vi "Lab Panel V5.27.vi"() -> ()   [LabVIEW 2013] (continued)
                            n1774 = Bundle(cluster=w3324) -> (w3325:T4)  [unwired: 3 in]
                            n1775 = local write "RUN LAB05-2"(w3322) -> ()
                            n1776 = local write "O/I  LAB05-2"(w3322) -> ()
                            n1777 = local write "run lab05-2"(w3322) -> ()
                            n1778 = local write "DISP LAB05-2"(w3325) -> ()
                          }
                          frame #1 {
                            n1779 = TDMS Close(11:w3326) -> (0:w3327:errorcluster)  [unwired: 1 in, 1 out]
                            n1780 = local write "data file error"(w3327) -> ()
                          }
                          frame #2 {
                            n1781 = stacked-sequence {
                              tunnel: "LAB05-2" -> [w3335 w3341]
                              tunnel: w3332 -> [_ w3340]
                              tunnel: w3331 -> [_ w3339]
                              tunnel: w3330 -> [_ w3338]
                              tunnel: w3329 -> [_ w3337]
                              tunnel: w3328 -> [_ w3336]
                              frame #0 {
                                n1782 = call "sub vi - defrag tdms v1.vi"("panel id"=w3335) -> ("error out"=w3334:errorcluster)  [unwired: 10 in]
                                n1783 = local write "data file error"(w3334) -> ()
                              }
                              frame #1 {
                                n1784 = Bundle("STATUS"=w3340, "OUT SERVER ADDRESS"=w3339, "FROM ACCOUNT"=w3338, "Mail Test File To:"=w3337, "Mail Test Fail"=w3336) -> (w3343:T26)  [unwired: 1 in]
                                n1785 = call "Save data file (pass-fail) v5.vi"("Input Cluster"=w3343, "panel id"=w3341) -> ("network file save error"=w3342:errorcluster)  [unwired: 8 in, 1 out]
                                n1786 = local write "data file error"(w3342) -> ()
                              }
                            }
                          }
                        }
                      }
                    }
                  }
                }
              }
            }
            n1787 = global write "Global display 2.vi" "Mail test file to:"(w2851) -> ()
            n1788 = local read "Network Directory"() -> (w2857:path)
            n1789 = global write "Global 1.vi" "Network Drive"(w2857) -> ()
          }
          frame #8 {
            # "disable functions"
            n1790 = stacked-sequence {
              tunnel: w3353 -> [w3367 _ w3424]
              tunnel: w3352 -> [w3362 _ w3423]
              tunnel: w3351 -> [w3361 _ w3422]
              tunnel: w3350 -> [w3359 _ w3421]
              tunnel: w3349 -> [w3360 _ w3420]
              tunnel: w3348 -> [_ w3384 w3419]
              tunnel: w3347 -> [_ w3385 w3418]
              tunnel: w3346 -> [_ w3386 w3417]
              tunnel: w3345 -> [_ w3387 w3416]
              tunnel: w3344 -> [_ w3388 w3415]
              frame #0 {
                n1791 = Select(t=2, s=w3359, f=0) -> (s? t:f=w3355:i32)
                n1792 = Select(t=2, s=w3361, f=0) -> (s? t:f=w3356:i32)
                n1793 = Select(t=2, s=w3360, f=0) -> (s? t:f=w3354:i32)
                n1794 = Select(t=2, s=w3367, f=0) -> (s? t:f=w3358:i32)
                n1795 = Select(t=2, s=w3362, f=0) -> (s? t:f=w3357:i32)
                n1796 = property on="SELECT LAB02-2" class="RadioBtnsControl (strict)"("DisabledEnum"=w3355) -> ()  [unwired: 2 in, 2 out]
                n1797 = property on="SELECT LAB02-1" class="RadioBtnsControl (strict)"("DisabledEnum"=w3356) -> ()  [unwired: 2 in, 2 out]
                n1798 = property on="SELECT LAB03-1" class="RadioBtnsControl (strict)"("DisabledEnum"=w3354) -> ()  [unwired: 2 in, 2 out]
                n1799 = property on="SELECT LAB01-1" class="RadioBtnsControl (strict)"("DisabledEnum"=w3358) -> ()  [unwired: 2 in, 2 out]
                n1800 = property on="SELECT LAB01-2" class="RadioBtnsControl (strict)"("DisabledEnum"=w3357) -> ()  [unwired: 2 in, 2 out]
                n1801 = Not(x=w3367) -> (.not. x?=w3368:bool)
                n1802 = property on="RESULT LAB01-1" class="Bool (strict)"("Visible"=w3368) -> ()  [unwired: 2 in, 2 out]
                n1803 = Not(x=w3362) -> (.not. x?=w3366:bool)
                n1804 = Not(x=w3361) -> (.not. x?=w3365:bool)
                n1805 = Not(x=w3359) -> (.not. x?=w3364:bool)
                n1806 = property on="RESULT LAB01-2" class="Bool (strict)"("Visible"=w3366) -> ()  [unwired: 2 in, 2 out]
                n1807 = Not(x=w3360) -> (.not. x?=w3363:bool)
                n1808 = property on="RESULT LAB02-1" class="Bool (strict)"("Visible"=w3365) -> ()  [unwired: 2 in, 2 out]
                n1809 = property on="RESULT LAB02-2" class="Bool (strict)"("Visible"=w3364) -> ()  [unwired: 2 in, 2 out]
                n1810 = property on="RESULT LAB03-1" class="Bool (strict)"("Visible"=w3363) -> ()  [unwired: 2 in, 2 out]
                n1811 = property on="SET LAB01-1" class="Clust (strict)"("DisabledEnum"=w3358) -> ()  [unwired: 2 in, 2 out]
                n1812 = property on="SET LAB01-2" class="Clust (strict)"("DisabledEnum"=w3357) -> ()  [unwired: 2 in, 2 out]
                n1813 = property on="SET LAB02-1" class="Clust (strict)"("DisabledEnum"=w3356) -> ()  [unwired: 2 in, 2 out]
                n1814 = property on="SET LAB02-2" class="Clust (strict)"("DisabledEnum"=w3355) -> ()  [unwired: 2 in, 2 out]
                n1815 = property on="SET LAB03-1" class="Clust (strict)"("DisabledEnum"=w3354) -> ()  [unwired: 2 in, 2 out]
                n1816 = property on="O/I  LAB01-1" class="Bool (strict)"("DisabledEnum"=w3358) -> ()  [unwired: 2 in, 2 out]
                n1817 = property on="O/I  LAB01-2" class="Bool (strict)"("DisabledEnum"=w3357) -> ()  [unwired: 2 in, 2 out]
                n1818 = property on="O/I  LAB02-1" class="Bool (strict)"("DisabledEnum"=w3356) -> ()  [unwired: 2 in, 2 out]
                n1819 = property on="O/I  LAB02-2" class="Bool (strict)"("DisabledEnum"=w3355) -> ()  [unwired: 2 in, 2 out]
                n1820 = property on="O/I  LAB03-1" class="Bool (strict)"("DisabledEnum"=w3354) -> ()  [unwired: 2 in, 2 out]
              }
              frame #1 {
                n1821 = Select(t=2, s=w3388, f=0) -> (s? t:f=w3379:i32)
                n1822 = Select(t=2, s=w3387, f=0) -> (s? t:f=w3380:i32)
                n1823 = Select(t=2, s=w3384, f=0) -> (s? t:f=w3383:i32)
                n1824 = Select(t=2, s=w3385, f=0) -> (s? t:f=w3382:i32)
                n1825 = Select(t=2, s=w3386, f=0) -> (s? t:f=w3381:i32)
                n1826 = property on="SELECT LAB05-2" class="RadioBtnsControl (strict)"("DisabledEnum"=w3379) -> ()  [unwired: 2 in, 2 out]
                n1827 = property on="SELECT LAB05-1" class="RadioBtnsControl (strict)"("DisabledEnum"=w3380) -> ()  [unwired: 2 in, 2 out]
                n1828 = property on="SELECT LAB03-2" class="RadioBtnsControl (strict)"("DisabledEnum"=w3383) -> ()  [unwired: 2 in, 2 out]
                n1829 = property on="SELECT LAB04-1" class="RadioBtnsControl (strict)"("DisabledEnum"=w3382) -> ()  [unwired: 2 in, 2 out]
                n1830 = property on="SELECT LAB04-2" class="RadioBtnsControl (strict)"("DisabledEnum"=w3381) -> ()  [unwired: 2 in, 2 out]
                n1831 = property on="SET LAB05-2" class="Clust (strict)"("DisabledEnum"=w3379) -> ()  [unwired: 2 in, 2 out]
                n1832 = property on="SET LAB05-1" class="Clust (strict)"("DisabledEnum"=w3380) -> ()  [unwired: 2 in, 2 out]
                n1833 = property on="SET LAB03-2" class="Clust (strict)"("DisabledEnum"=w3383) -> ()  [unwired: 2 in, 2 out]
                n1834 = property on="SET LAB04-1" class="Clust (strict)"("DisabledEnum"=w3382) -> ()  [unwired: 2 in, 2 out]
                n1835 = property on="SET LAB04-2" class="Clust (strict)"("DisabledEnum"=w3381) -> ()  [unwired: 2 in, 2 out]
                n1836 = property on="O/I  LAB05-2" class="Bool (strict)"("DisabledEnum"=w3379) -> ()  [unwired: 2 in, 2 out]
                n1837 = property on="O/I  LAB05-1" class="Bool (strict)"("DisabledEnum"=w3380) -> ()  [unwired: 2 in, 2 out]
                n1838 = property on="O/I  LAB04-1" class="Bool (strict)"("DisabledEnum"=w3382) -> ()  [unwired: 2 in, 2 out]
                n1839 = property on="O/I  LAB04-2" class="Bool (strict)"("DisabledEnum"=w3381) -> ()  [unwired: 2 in, 2 out]
                n1840 = property on="O/I  LAB03-2" class="Bool (strict)"("DisabledEnum"=w3383) -> ()  [unwired: 2 in, 2 out]
                n1841 = Not(x=w3388) -> (.not. x?=w3389:bool)
                n1842 = Not(x=w3387) -> (.not. x?=w3390:bool)
                n1843 = Not(x=w3386) -> (.not. x?=w3391:bool)
                n1844 = property on="RESULT LAB05-2" class="Bool (strict)"("Visible"=w3389) -> ()  [unwired: 2 in, 2 out]
                n1845 = property on="RESULT LAB05-1" class="Bool (strict)"("Visible"=w3390) -> ()  [unwired: 2 in, 2 out]
                n1846 = Not(x=w3385) -> (.not. x?=w3392:bool)
                n1847 = property on="RESULT LAB04-2" class="Bool (strict)"("Visible"=w3391) -> ()  [unwired: 2 in, 2 out]
                n1848 = Not(x=w3384) -> (.not. x?=w3393:bool)
                n1849 = property on="RESULT LAB04-1" class="Bool (strict)"("Visible"=w3392) -> ()  [unwired: 2 in, 2 out]
                n1850 = property on="RESULT LAB03-2" class="Bool (strict)"("Visible"=w3393) -> ()  [unwired: 2 in, 2 out]
              }
              frame #2 {
                # "disable calibrate if any test running"
                n1851 = Or(x=w3416, y=w3415) -> (x .or. y?=w3409:bool)
                n1852 = Or(x=w3418, y=w3417) -> (x .or. y?=w3411:bool)
                n1853 = Or(x=w3422, y=w3421) -> (x .or. y?=w3413:bool)
                n1854 = Or(x=w3420, y=w3419) -> (x .or. y?=w3412:bool)
                n1855 = Or(x=w3424, y=w3423) -> (x .or. y?=w3414:bool)
                n1856 = Or(x=w3412, y=w3411) -> (x .or. y?=w3410:bool)
                n1857 = Or(x=w3414, y=w3413) -> (x .or. y?=w3408:bool)
                n1858 = Or(x=w3410, y=w3409) -> (x .or. y?=w3407:bool)
                n1859 = Or(x=w3408, y=w3407) -> (x .or. y?=w3404:bool)
                "Any Test Running" <- w3404
                n1860 = case shown="False" w3404 {
                  tunnel: [0 2] -> w3406
                  frame False {
                  }
                  frame True {
                  }
                }
                n1861 = property on="JIG TEST" class="Clust (strict)"("DisabledEnum"=w3406) -> ()  [unwired: 2 in, 2 out]
                n1862 = property on="Network Directory" class="Path"("DisabledEnum"=w3406) -> ()  [unwired: 2 in, 2 out]
                n1863 = property on="MAIL SETTINGS" class="Clust (strict)"("DisabledEnum"=w3406) -> ()  [unwired: 2 in, 2 out]
                n1864 = property on="SET (cal)" class="Bool (strict)"("DisabledEnum"=w3406) -> ()  [unwired: 2 in, 2 out]
                n1865 = property on="ADMIN" class="Bool (strict)"("DisabledEnum"=0) -> ()  [unwired: 2 in, 2 out]
              }
            }
          }
          frame #9 {
            # "drive jigs"
            n1866 = stacked-sequence {
              frame #0 {
                # "jig on"
                n1867 = local read "jig cycle"() -> (w3432:dbl)
                n1868 = property on="JIG TEST" class="Clust (strict)"() -> ("DisabledEnum"=w3429:T16)  [unwired: 2 in, 2 out]
                n1869 = Equal?(x=w3429, y=2) -> (x = y?=w3428:bool)
                n1870 = Equal?(x=w3432, y=0) -> (x = y?=w3430:bool)
                n1871 = And(x=w3430, y=w3428) -> (x .and. y?=w3427:bool)
                n1872 = case shown="True" w3427 {
                  frame False {
                  }
                  frame True {
                    n1873 = local read "run lab01-1"() -> (w3443:bool)
                    n1874 = local read "run lab01-2"() -> (w3442:bool)
                    n1875 = local read "run lab02-1"() -> (w3441:bool)
                    n1876 = local read "run lab02-2"() -> (w3440:bool)
                    n1877 = local read "run lab03-1"() -> (w3439:bool)
                    n1878 = local read "run lab03-2"() -> (w3438:bool)
                    n1879 = local read "run lab04-1"() -> (w3437:bool)
                    n1880 = local read "run lab04-2"() -> (w3436:bool)
                    n1881 = local read "run lab05-1"() -> (w3435:bool)
                    n1882 = local read "run lab05-2"() -> (w3434:bool)
                    n1883 = local write "JIG LAB03-2"(w3438) -> ()
                    n1884 = local write "JIG LAB01-1"(w3443) -> ()
                    n1885 = local write "JIG LAB01-2"(w3442) -> ()
                    n1886 = local write "JIG LAB02-1"(w3441) -> ()
                    n1887 = local write "JIG LAB02-2"(w3440) -> ()
                    n1888 = local write "JIG LAB03-1"(w3439) -> ()
                    n1889 = local write "JIG LAB04-1"(w3437) -> ()
                    n1890 = local write "JIG LAB04-2"(w3436) -> ()
                    n1891 = local write "JIG LAB05-1"(w3435) -> ()
                    n1892 = local write "JIG LAB05-2"(w3434) -> ()
                  }
                }
              }
              frame #1 {
                # "jig off"
                n1893 = local read "jig cycle"() -> (w3450:dbl)
                n1894 = local read "on loops"() -> (w3449:dbl)
                n1895 = property on="JIG TEST" class="Clust (strict)"() -> ("DisabledEnum"=w3448:T16)  [unwired: 2 in, 2 out]
                n1896 = Equal?(x=w3448, y=2) -> (x = y?=w3446:bool)
                n1897 = Equal?(x=w3450, y=w3449) -> (x = y?=w3445:bool)
                n1898 = And(x=w3445, y=w3446) -> (x .and. y?=w3444:bool)
                n1899 = case shown="True" w3444 {
                  frame False {
                  }
                  frame True {
                    w3501 = FALSE
                    w3502 = TRUE
                    w3500 = 2
                    n1900 = local read "SELECT LAB05-2"() -> (w3491:T3)
                    n1901 = local read "SELECT LAB04-2"() -> (w3493:T3)
                    n1902 = local read "SELECT LAB04-1"() -> (w3494:T3)
                    n1903 = local read "SELECT LAB05-1"() -> (w3492:T3)
                    n1904 = local read "SELECT LAB03-2"() -> (w3495:T3)
                    n1905 = local read "SELECT LAB02-1"() -> (w3498:T3)
                    n1906 = local read "SELECT LAB03-1"() -> (w3496:T3)
                    n1907 = local read "SELECT LAB02-2"() -> (w3497:T3)
                    n1908 = local read "SELECT LAB01-2"() -> (w3499:T3)
                    n1909 = local read "run lab05-1"() -> (w3461:bool)
                    n1910 = local read "run lab05-2"() -> (w3460:bool)
                    n1911 = local read "SELECT LAB01-1"() -> (w3503:T3)
                    n1912 = local read "run lab04-2"() -> (w3462:bool)
                    n1913 = local read "run lab04-1"() -> (w3463:bool)
                    n1914 = local read "run lab01-1"() -> (w3479:bool)
                    n1915 = local read "run lab01-2"() -> (w3468:bool)
                    n1916 = local read "run lab03-2"() -> (w3464:bool)
                    n1917 = local read "run lab03-1"() -> (w3465:bool)
                    n1918 = local read "run lab02-1"() -> (w3467:bool)
                    n1919 = local read "run lab02-2"() -> (w3466:bool)
                    n1920 = Equal?(x=w3500, y=w3496) -> (x = y?=w3474:bool)
                    n1921 = Equal?(x=w3500, y=w3495) -> (x = y?=w3473:bool)
                    n1922 = Equal?(x=w3500, y=w3494) -> (x = y?=w3472:bool)
                    n1923 = Equal?(x=w3500, y=w3493) -> (x = y?=w3471:bool)
                    n1924 = Equal?(x=w3500, y=w3492) -> (x = y?=w3470:bool)
                    n1925 = Equal?(x=w3500, y=w3491) -> (x = y?=w3469:bool)
                    n1926 = Equal?(x=w3500, y=w3503) -> (x = y?=w3480:bool)
                    n1927 = Equal?(x=w3500, y=w3498) -> (x = y?=w3476:bool)
                    n1928 = Equal?(x=w3500, y=w3497) -> (x = y?=w3475:bool)
                    n1929 = Equal?(x=w3500, y=w3499) -> (x = y?=w3477:bool)
                    n1930 = And(x=w3471, y=w3462) -> (x .and. y?=w3453:bool)
                    n1931 = And(x=w3474, y=w3465) -> (x .and. y?=w3456:bool)
                    n1932 = And(x=w3472, y=w3463) -> (x .and. y?=w3454:bool)
                    n1933 = And(x=w3469, y=w3460) -> (x .and. y?=w3451:bool)
                    n1934 = And(x=w3475, y=w3466) -> (x .and. y?=w3457:bool)
                    n1935 = And(x=w3473, y=w3464) -> (x .and. y?=w3455:bool)
                    n1936 = And(x=w3470, y=w3461) -> (x .and. y?=w3452:bool)
                    n1937 = And(x=w3477, y=w3468) -> (x .and. y?=w3459:bool)
                    n1938 = And(x=w3480, y=w3479) -> (x .and. y?=w3478:bool)
                    n1939 = And(x=w3476, y=w3467) -> (x .and. y?=w3458:bool)
                    n1940 = Select(t=w3502, s=w3478, f=w3501) -> (s? t:f=w3481:bool)
                    n1941 = Select(t=w3502, s=w3459, f=w3501) -> (s? t:f=w3482:bool)
                    n1942 = Select(t=w3502, s=w3458, f=w3501) -> (s? t:f=w3483:bool)
                    n1943 = Select(t=w3502, s=w3457, f=w3501) -> (s? t:f=w3484:bool)
                    n1944 = Select(t=w3502, s=w3456, f=w3501) -> (s? t:f=w3485:bool)
                    n1945 = Select(t=w3502, s=w3455, f=w3501) -> (s? t:f=w3486:bool)
                    n1946 = Select(t=w3502, s=w3454, f=w3501) -> (s? t:f=w3487:bool)
                    n1947 = Select(t=w3502, s=w3453, f=w3501) -> (s? t:f=w3488:bool)
                    n1948 = Select(t=w3502, s=w3452, f=w3501) -> (s? t:f=w3489:bool)
                    n1949 = Select(t=w3502, s=w3451, f=w3501) -> (s? t:f=w3490:bool)
                    n1950 = local write "JIG LAB03-2"(w3486) -> ()
                    n1951 = local write "JIG LAB02-1"(w3483) -> ()
                    n1952 = local write "JIG LAB02-2"(w3484) -> ()
                    n1953 = local write "JIG LAB01-2"(w3482) -> ()
                    n1954 = local write "JIG LAB03-1"(w3485) -> ()
                    n1955 = local write "JIG LAB01-1"(w3481) -> ()
                    n1956 = local write "JIG LAB05-2"(w3490) -> ()
                    n1957 = local write "JIG LAB04-1"(w3487) -> ()
                    n1958 = local write "JIG LAB05-1"(w3489) -> ()
                    n1959 = local write "JIG LAB04-2"(w3488) -> ()
                  }
                }
              }
            }
          }
          frame #10 {
            # "enable  jig test output if no test busy"
            n1960 = property on="JIG TEST" class="Clust (strict)"() -> ("DisabledEnum"=w3506:T16)  [unwired: 2 in, 2 out]
            n1961 = Equal?(x=w3506, y=0) -> (x = y?=w3504:bool)
            n1962 = case shown="True" w3504 {
              frame False {
              }
              frame True {
                n1963 = local read "JIG TEST"() -> (w3517:T10)
                n1964 = Unbundle(w3517) -> ("LAB01-1"=w3516:bool, "LAB01-2"=w3515:bool, "LAB02-1"=w3514:bool, "LAB02-2"=w3513:bool, "LAB03-1"=w3512:bool, "LAB03-2"=w3511:bool, "LAB04-1"=w3510:bool, "LAB04-2"=w3509:bool, "LAB05-1"=w3508:bool, "LAB05-2"=w3507:bool)
                n1965 = local write "JIG LAB05-1"(w3508) -> ()
                n1966 = local write "JIG LAB05-2"(w3507) -> ()
                n1967 = local write "JIG LAB04-1"(w3510) -> ()
                n1968 = local write "JIG LAB04-2"(w3509) -> ()
                n1969 = local write "JIG LAB03-2"(w3511) -> ()
                n1970 = local write "JIG LAB01-1"(w3516) -> ()
                n1971 = local write "JIG LAB02-1"(w3514) -> ()
                n1972 = local write "JIG LAB03-1"(w3512) -> ()
                n1973 = local write "JIG LAB01-2"(w3515) -> ()
                n1974 = local write "JIG LAB02-2"(w3513) -> ()
              }
            }
          }
          frame #11 {
            w3518 = FALSE
            # "Drive digital output and reset USB and temperature network if required."
            n1975 = global read "Global display 3.vi" "cycle O/F"() -> (w3527:bool)
            n1976 = local read "O/I  LAB05-2"() -> (w3520:bool)
            n1977 = local read "O/I  LAB05-1"() -> (w3522:bool)
            n1978 = local read "JIG LAB05-2"() -> (w3519:bool)
            n1979 = local read "O/I  LAB04-2"() -> (w3524:bool)
            n1980 = local read "JIG LAB05-1"() -> (w3521:bool)
            n1981 = local read "JIG LAB04-2"() -> (w3523:bool)
            n1982 = local read "O/I  LAB03-1"() -> (w3538:bool)
            n1983 = local read "O/I  LAB04-1"() -> (w3534:bool)
            n1984 = local read "O/I  LAB02-1"() -> (w3542:bool)
            n1985 = local read "O/I  LAB02-2"() -> (w3540:bool)
            n1986 = local read "O/I  LAB03-2"() -> (w3536:bool)
            n1987 = local read "JIG LAB04-1"() -> (w3533:bool)
            n1988 = local read "JIG LAB03-2"() -> (w3535:bool)
            n1989 = local read "O/I  LAB01-2"() -> (w3544:bool)
            n1990 = local read "JIG LAB02-1"() -> (w3541:bool)
            n1991 = local read "JIG LAB02-2"() -> (w3539:bool)
            n1992 = local read "JIG LAB03-1"() -> (w3537:bool)
            n1993 = local read "O/I  LAB01-1"() -> (w3546:bool)
            n1994 = local read "JIG LAB01-2"() -> (w3543:bool)
            n1995 = local read "JIG LAB01-1"() -> (w3545:bool)
            n1996 = case shown="False" w3527 {
              tunnel: [w3662 FALSE] -> w3526
              frame False {
                n1997 = local read "Analog error"() -> (w3664:bool)
                n1998 = local read "Reset Measuring"() -> (w3663:bool)
                n1999 = Or(x=w3663, y=w3664) -> (x .or. y?=w3662:bool)
              }
              frame True {
              }
            }
            n2000 = Build Array(w3539, w3538, w3537, w3536, w3535, w3534, w3533) -> (w3531:bool[])
            "USB OUT 1" <- w3531
            n2001 = Build Array(w3546, w3545, w3544, w3543, w3542, w3541, w3540) -> (w3532:bool[])
            "USB OUT 0" <- w3532
            n2002 = Build Array(w3524, w3523, w3522, w3521, w3520, w3519, w3518, w3518) -> (w3530:bool[])
            "USB OUT 2" <- w3530
            n2003 = Not(x=w3527) -> (.not. x?=w3528:bool)
            n2004 = local read "Simulate"() -> (w3529:bool)
            n2005 = And(x=w3528, y=w3526) -> (x .and. y?=w3525:bool)
            n2006 = stacked-sequence {
              tunnel: w3532 -> [w3550 w3556]
              tunnel: w3531 -> [w3549 w3555]
              tunnel: w3530 -> [w3548 w3554]
              tunnel: w3529 -> [w3547 w3557]
              tunnel: w3525 -> [_ w3558]
              frame #0 {
                # "drive outputs for normal use"
                n2007 = case shown="False" w3547 {
                  tunnel: w3550 -> [w3553 _]
                  tunnel: w3549 -> [w3552 _]
                  tunnel: w3548 -> [w3551 _]
                  frame False {
                    n2008 = call "sub vi - Drive Relays All v6.vi"("Array #2"=w3551, "Array #1"=w3552, "Array #0"=w3553) -> ()  [unwired: 8 in, 1 out]
                  }
                  frame True {
                  }
                }
              }
              frame #1 {
                # "USB  reset routine"
                n2009 = case shown="True" w3558 {
                  tunnel: w3557 -> [_ w3562]
                  tunnel: w3556 -> [_ w3561]
                  tunnel: w3555 -> [_ w3560]
                  tunnel: w3554 -> [_ w3559]
                  frame False {
                  }
                  frame True {
                    n2010 = stacked-sequence {
                      seq-local: [w3564 _ _ _ _] -> [_ w3570 _ _ _]
                      tunnel: w3562 -> [_ w3574 _ _ _]
                      tunnel: w3561 -> [_ w3573 _ _ _]
                      tunnel: w3560 -> [_ w3572 _ _ _]
                      tunnel: w3559 -> [_ w3571 _ _ _]
                      frame #0 {
                        n2011 = case shown="False" "Auto Reset" {
                          tunnel: [w3567 FALSE] -> w3565
                          frame False {
                            n2012 = Two Button Dialog(message="System reset") -> (T button?=w3567:bool)  [unwired: 2 in]
                          }
                          frame True {
                          }
                        }
                        n2013 = disable-structure shown="Disabled" {
                          frame Disabled {
                            n2014 = local write "Tab Control 2"(5) -> ()
                          }
                          frame Enabled {
                          }
                        }
                        n2015 = Or(x="Auto Reset", y=w3565) -> (x .or. y?=w3564:bool)
                      }
                      frame #1 {
                        n2016 = case shown="True" w3570 {
                          tunnel: w3574 -> [_ w3580]
                          tunnel: w3573 -> [_ w3579]
                          tunnel: w3572 -> [_ w3578]
                          tunnel: w3571 -> [_ w3577]
                          frame False {
                          }
                          frame True {
                            n2017 = stacked-sequence {
                              tunnel: w3580 -> [_ w3598 _]
                              tunnel: bool[] [] -> [w3583 w3597 w3619]
                              tunnel: w3579 -> [_ _ w3618]
                              tunnel: w3578 -> [w3582 _ w3617]
                              tunnel: w3577 -> [w3581 _ w3616]
                              tunnel: 5000 -> [w3584 _ w3615]
                              frame #0 {
                                # "switch off test stations for system reset"
                                n2018 = stacked-sequence {
                                tunnel: w3584 -> [w3588 w3592 w3594]
                                tunnel: w3583 -> [w3587 w3591 w3595]
                                tunnel: w3582 -> [w3586 _ _]
                                tunnel: w3581 -> [w3585 w3590 _]
                                frame #0 {
                                # "drive 1st 7 inputs"
                                n2019 = call "sub vi - Drive Relays All v6.vi"("Array #2"=w3585, "Array #1"=w3586, "Array #0"=w3587) -> ()  [unwired: 8 in, 1 out]
                                n2020 = call "Message Display V1.vi"("Message"="Delay off LAB 01-1 to 02-1", "Delay mS"=w3588) -> ()  [unwired: 10 in]
                                }
                                frame #1 {
                                # "drive 2nd 7 inputs"
                                n2021 = call "sub vi - Drive Relays All v6.vi"("Array #2"=w3590, "Array #1"=w3591, "Array #0"=w3591) -> ()  [unwired: 8 in, 1 out]
                                n2022 = call "Message Display V1.vi"("Message"="Delay off LAB 02-2 to 04-1", "Delay mS"=w3592) -> ()  [unwired: 10 in]
                                }
                                frame #2 {
                                # "drive 3rd 7 inputs"
                                n2023 = call "sub vi - Drive Relays All v6.vi"("Array #2"=w3595, "Array #1"=w3595, "Array #0"=w3595) -> ()  [unwired: 8 in, 1 out]
                                n2024 = call "Message Display V1.vi"("Message"="Delay off LAB 04-2 to 05-2", "Delay mS"=w3594) -> ()  [unwired: 10 in]
                                }
                                }
                              }
                              frame #1 {
                                # "reset all usb modules"
                                n2025 = stacked-sequence {
                                tunnel: w3598 -> [_ w3603]
                                tunnel: w3597 -> [w3601 _]
                                frame #0 {
                                n2026 = local write "AI Task"(FALSE) -> ()
                                n2027 = call "sub vi - Drive Relays All v6.vi"("Array #2"=bool[] [FALSE, FALSE, FALSE, FALSE, FALSE, FALSE, TRUE, FALSE], "Array #1"=w3601, "Array #0"=w3601) -> ()  [unwired: 8 in, 1 out]
                                }
                                frame #1 {
                                n2028 = call "Reset Meas v 5.vi"("simulate"=w3603) -> ("Reset Error"=w3602:bool)  [unwired: 10 in]
                                n2029 = case shown="False" w3602 {
                                frame False {
                                n2030 = local read "AI Task0"() -> (w3610:dbl)
                                n2031 = local read "AI Task1"() -> (w3609:dbl)
                                n2032 = local read "AI Task2"() -> (w3608:dbl)
                                n2033 = local read "RATE (Hz)"() -> (w3607:dbl)
                                n2034 = local read "SAMPLES"() -> (w3606:dbl)
                                n2035 = call "sub vi - AI USB4704 (3)  Create Task v3.vi"("Task In 0"=w3610, "Task In 1"=w3609, "Task In 2"=w3608, "Rate Hz"=w3607, "Samples"=w3606) -> ("TASK USB 0"=w3613:i32, "TASK USB 1"=w3612:i32, "TASK USB 2"=w3611:i32, "AI Task Er"=w3604:bool)  [unwired: 6 in, 1 out]
                                n2036 = local write "AI Task"(TRUE) -> ()
                                n2037 = local write "Reset Error"(w3604) -> ()
                                n2038 = local write "AI Task2"(w3611) -> ()
                                n2039 = local write "AI Task1"(w3612) -> ()
                                n2040 = local write "AI Task0"(w3613) -> ()
                                }
                                frame True {
                                "Reset Error" <- TRUE
                                }
                                }
                                }
                                }
                              }
                              frame #2 {
                                # "switch test stations back on after reset"
                                n2041 = stacked-sequence {
                                tunnel: w3619 -> [w3623 w3626 _]
                                tunnel: w3618 -> [w3622 w3628 w3633]
                                tunnel: w3615 -> [w3621 w3624 w3630]
                                tunnel: w3617 -> [_ w3627 w3632]
                                tunnel: w3616 -> [_ _ w3629]
                                frame #0 {
                                # "drive 1st 7 inputs"
                                n2042 = call "sub vi - Drive Relays All v6.vi"("Array #2"=w3623, "Array #1"=w3623, "Array #0"=w3622) -> ()  [unwired: 8 in, 1 out]
                                n2043 = call "Message Display V1.vi"("Message"="Delay on LAB 01-1 to 02-1", "Delay mS"=w3621) -> ()  [unwired: 10 in]
                                }
                                frame #1 {
                                # "drive 1st & 2nd outputs"
                                n2044 = call "sub vi - Drive Relays All v6.vi"("Array #2"=w3626, "Array #1"=w3627, "Array #0"=w3628) -> ()  [unwired: 8 in, 1 out]
                                n2045 = call "Message Display V1.vi"("Message"="Delay on LAB 02-2 to 04-1", "Delay mS"=w3624) -> ()  [unwired: 10 in]
                                }
                                frame #2 {
                                n2046 = call "sub vi - Drive Relays All v6.vi"("Array #2"=w3629, "Array #1"=w3632, "Array #0"=w3633) -> ()  [unwired: 8 in, 1 out]
                                n2047 = call "Message Display V1.vi"("Message"="Delay on LAB 04-2 to 05-2", "Delay mS"=w3630) -> ()  [unwired: 10 in]
                                }
                                }
                              }
                            }
                          }
                        }
                      }
                      frame #2 {
                        w3634 = 0
                        w3635 = FALSE
                        # "set all back to zero"
                        n2048 = local read "Total USB resets"() -> (w3637:dbl)
                        n2049 = local read "Resets Done"() -> (w3639:dbl)
                        n2050 = local write "Reset Measuring"(w3635) -> ()
                        n2051 = local write "Analog error"(w3635) -> ()
                        n2052 = local write "Er USB#2"(w3634) -> ()
                        n2053 = local write "Er USB#0"(w3634) -> ()
                        n2054 = local write "Er USB#1"(w3634) -> ()
                        n2055 = local write "Error USB #0"(w3635) -> ()
                        n2056 = local write "Error USB #1"(w3635) -> ()
                        n2057 = local write "Error USB #2"(w3635) -> ()
                        n2058 = Increment(x=w3637) -> (x+1=w3636:dbl)
                        n2059 = Increment(x=w3639) -> (x+1=→"Resets Done":dbl)
                        n2060 = local write "Total USB resets"(w3636) -> ()
                      }
                      frame #3 {
                        # "save reset value"
                        n2061 = String To Path(string="c:\\crabtree\\Set Up\\") -> (path=w3649:path)
                        n2062 = Build Path(base path=w3649, name or relative path="USB resets.bin") -> (appended path=w3642:path)
                        n2063 = Create Folder(path (use dialog)=w3649) -> (error out=w3641:errorcluster)  [unwired: 2 in, 2 out]
                        n2064 = local read "Total USB resets"() -> (w3640:dbl)
                        n2065 = call <vilib>:"Clear Errors.vi"("error in (no error)"=w3641) -> ()  [unwired: 6 in, 1 out]
                        n2066 = Open/Create/Replace File(file path (use dialog)=w3642, operation (0:open)=T17."replace or create") -> (refnum out=w3647:refnum<file>, error out=w3646:errorcluster)  [unwired: 4 in, 1 out]
                        n2067 = Write to Binary File(file (use dialog)=w3647, data=w3640, error in=w3646) -> (refnum out=w3645:refnum<file>, error out=w3644:errorcluster)  [unwired: 3 in, 1 out]
                        n2068 = Close File(refnum=w3645, error in=w3644) -> (error out=w3643:errorcluster)  [unwired: 1 out]
                        n2069 = local write "data file error"(w3643) -> ()
                      }
                      frame #4 {
                        # "mail reset value"
                        n2070 = local read "MAIL SETTINGS"() -> (w3655:T7)
                        n2071 = local read "Total USB resets"() -> (w3659:dbl)
                        n2072 = Unbundle(w3655) -> ("OUT SERVER ADDRESS"=w3661:string, "FROM ACCOUNT"=w3660:string)  [unwired: 5 out]
                        n2073 = Number To Decimal String(number=w3659) -> (decimal integer string=w3657:string)  [unwired: 1 in]
                        n2074 = Concatenate Strings("Total USB resets: ", w3657) -> (w3656:string)
                        n2075 = call "sub vi - send mail v5.vi"("TO:"="francois@ffg.net", "subject"=w3656, "from"=w3660, "out going server"=w3661) -> ("error out"=w3654:errorcluster)  [unwired: 11 in]
                        n2076 = Bundle(cluster=w3655, "mail error"=w3654) -> (w3653:T7)  [unwired: 6 in]
                        n2077 = local write "MAIL SETTINGS"(w3653) -> ()
                      }
                    }
                  }
                }
              }
            }
          }
          frame #12 {
            # "if all test panels are off stop analog read"
            n2078 = local read "O/I  LAB03-1"() -> (w3687:bool)
            n2079 = local read "O/I  LAB03-2"() -> (w3686:bool)
            n2080 = local read "O/I  LAB04-1"() -> (w3685:bool)
            n2081 = local read "O/I  LAB04-2"() -> (w3684:bool)
            n2082 = local read "O/I  LAB05-1"() -> (w3683:bool)
            n2083 = local read "O/I  LAB05-2"() -> (w3682:bool)
            n2084 = local read "O/I  LAB02-2"() -> (w3688:bool)
            n2085 = local read "O/I  LAB02-1"() -> (w3689:bool)
            n2086 = local read "O/I  LAB01-2"() -> (w3690:bool)
            n2087 = local read "O/I  LAB01-1"() -> (w3691:bool)
            n2088 = Or(x=w3683, y=w3682) -> (x .or. y?=w3680:bool)
            n2089 = Or(x=w3685, y=w3684) -> (x .or. y?=w3681:bool)
            n2090 = Or(x=w3689, y=w3688) -> (x .or. y?=w3679:bool)
            n2091 = Or(x=w3687, y=w3686) -> (x .or. y?=w3677:bool)
            n2092 = Or(x=w3691, y=w3690) -> (x .or. y?=w3678:bool)
            n2093 = Or(x=w3681, y=w3680) -> (x .or. y?=w3674:bool)
            n2094 = Or(x=w3678, y=w3679) -> (x .or. y?=w3676:bool)
            n2095 = Or(x=w3676, y=w3677) -> (x .or. y?=w3675:bool)
            n2096 = local read "Any Test Running"() -> (w3673:bool)
            n2097 = Or(x=w3675, y=w3674) -> (x .or. y?=w3672:bool)
            n2098 = local read "AI Task"() -> (w3668:bool)
            n2099 = Or(x=w3672, y=w3673) -> (x .or. y?=w3667:bool)
            n2100 = Not(x=w3667) -> (.not. x?=w3671:bool)
            n2101 = Not(x=w3668) -> (.not. x?=w3669:bool)
            n2102 = And(x=w3671, y=w3668) -> (x .and. y?=w3670:bool)
            n2103 = And(x=w3667, y=w3669) -> (x .and. y?=w3666:bool)
            n2104 = case shown="True" w3670 {
              frame False {
              }
              frame True {
                # "close task if no test"
                n2105 = stacked-sequence {
                  seq-local: [w3705 _] -> [_ w3716]
                  frame #0 {
                    # "send mail of test cycle values"
                    n2106 = local read "JIG RELAY CYCLES"() -> (w3709:T8)
                    n2107 = Cluster To Array(cluster=w3709) -> (array=w3706:dbl[])
                    n2108 = Reverse 1D Array(array=w3706) -> (reversed array=w3707:dbl[])
                    n2109 = for {
                      tunnel: w3707 -> [w3714] mode=indexing
                      shift-right: [w3712] -> w3705
                      shift-left: "" -> [w3711]
                      n2110 = Number To Decimal String(number=w3714) -> (decimal integer string=w3713:string)  [unwired: 1 in]
                      n2111 = Concatenate Strings(w3713, ":", w3711) -> (w3712:string)
                    }
                  }
                  frame #1 {
                    n2112 = local read "MAIL SETTINGS"() -> (w3718:T7)
                    n2113 = Unbundle(w3718) -> ("OUT SERVER ADDRESS"=w3719:string, "FROM ACCOUNT"=w3720:string)  [unwired: 5 out]
                    n2114 = Concatenate Strings("Test Cycles:", w3716) -> (w3722:string)
                    n2115 = call "sub vi - send mail v5.vi"("TO:"="francois@ffg.net", "subject"=w3722, "Info"="Jig total cycle values", "from"=w3720, "out going server"=w3719) -> ("error out"=w3723:errorcluster)  [unwired: 10 in]
                    n2116 = Bundle(cluster=w3718, "mail error"=w3723) -> (w3717:T7)  [unwired: 6 in]
                    n2117 = local write "MAIL SETTINGS"(w3717) -> ()
                  }
                }
                n2118 = local read "AI Task2"() -> (w3704:dbl)
                n2119 = local read "AI Task1"() -> (w3703:dbl)
                n2120 = local read "AI Task0"() -> (w3702:dbl)
                n2121 = local write "AI Task"(FALSE) -> ()
                n2122 = call "sub vi - AI USB4704 (3)  Close Task v1.vi"("TASK USB 0"=w3702, "TASK USB 1"=w3703, "TASK USB 2"=w3704) -> ()  [unwired: 13 in]
              }
            }
            n2123 = case shown="True" w3666 {
              frame False {
              }
              frame True {
                # "create task for test"
                n2124 = local read "SAMPLES"() -> (w3696:dbl)
                n2125 = local read "RATE (Hz)"() -> (w3695:dbl)
                n2126 = local read "AI Task2"() -> (w3694:dbl)
                n2127 = local read "AI Task0"() -> (w3692:dbl)
                n2128 = local read "AI Task1"() -> (w3693:dbl)
                n2129 = call "sub vi - AI USB4704 (3)  Create Task v3.vi"("Task In 0"=w3692, "Task In 1"=w3693, "Task In 2"=w3694, "Rate Hz"=w3695, "Samples"=w3696) -> ("TASK USB 0"=w3697:i32, "TASK USB 1"=w3698:i32, "TASK USB 2"=w3699:i32)  [unwired: 6 in, 2 out]
                n2130 = local write "AI Task0"(w3697) -> ()
                n2131 = local write "AI Task1"(w3698) -> ()
                n2132 = local write "AI Task2"(w3699) -> ()
                n2133 = local write "AI Task"(TRUE) -> ()
              }
            }
          }
          frame #13 {
            # "get all analog values from USB devices"
            n2134 = local read "on loops"() -> (w3732:dbl)
            n2135 = local read "jig cycle"() -> (w3729:dbl)
            n2136 = Add(x=w3732, y=3) -> (x+y=w3730:dbl)
            n2137 = Equal?(x=w3729, y=3) -> (x = y?=w3727:bool)
            n2138 = Equal?(x=w3729, y=w3730) -> (x = y?=w3728:bool)
            n2139 = Or(x=w3727, y=w3728) -> (x .or. y?=w3726:bool)
            n2140 = global write "Global display 3.vi" "cycle O/F"(w3727) -> ()
            n2141 = case shown="True" w3726 {
              tunnel: w3727 -> [_ w3738]
              tunnel: w3725 -> [_ w3735]
              frame False {
              }
              frame True {
                n2142 = local read "Simulate"() -> (w3741:bool)
                n2143 = case shown="False" w3741 {
                  tunnel: [w3757 dynamicdata[] [] ("array GRAPH")] -> w3747
                  tunnel: [w3756 w3782] -> w3746
                  tunnel: [w3755 w3782] -> w3745
                  tunnel: [w3754 w3782] -> w3744
                  tunnel: [w3753 w3782] -> w3743
                  tunnel: [w3752 w3782] -> w3742
                  tunnel: w3738 -> [_ w3786]
                  tunnel: [w3751 "Ambient Volts"] -> w3737
                  tunnel: [w3750 bool[] []] -> w3736
                  tunnel: w3735 -> [w3749 _]
                  tunnel: [w3748 0.3 ("Analog loop time")] -> w3734
                  frame False {
                    # "analog in"
                    n2144 = case shown="True" w3749 {
                      tunnel: [dynamicdata[] [] ("array GRAPH") w3776] -> w3757
                      tunnel: [w3759 w3775] -> w3756
                      tunnel: [w3759 w3774] -> w3755
                      tunnel: [w3759 w3773] -> w3754
                      tunnel: [w3759 w3772] -> w3753
                      tunnel: [w3759 w3771] -> w3752
                      tunnel: [3 w3770] -> w3751
                      tunnel: [bool[] [] w3769] -> w3750
                      tunnel: [0.0 w3765] -> w3748
                      frame False {
                        w3760 = 0.0
                        # "no test"
                        n2145 = Bundle(w3760, w3760, w3760, w3760, w3760, w3760) -> (w3759:cluster{dbl, dbl, dbl, dbl, dbl, dbl})  [unwired: 1 in]
                      }
                      frame True {
                        # "test on"
                        n2146 = local read "AI data 0"() -> (w3768:waveform(dbl)[])
                        n2147 = local read "AI data 1"() -> (w3767:waveform(dbl)[])
                        n2148 = local read "AI data 2"() -> (w3764:waveform(dbl)[])
                        n2149 = local read "AI Error"() -> (w3766:errorcluster[])
                        n2150 = call "sub vi - Read Analog All v9.5.vi"("data 0"=w3768, "data 1"=w3767, "data 2"=w3764, "AI Error"=w3766) -> ("array GRAPH"=w3776:dynamicdata[], "LAB01"=w3775:T27, "LAB02"=w3774:T28, "LAB03"=w3773:T29, "LAB04"=w3772:T30, "deg C"=w3770:dbl, "USB Error"=w3769:bool[], "LAB05"=w3771:T31)  [unwired: 4 in]
                        n2151 = local read "AI loop time"() -> (w3765:dbl)
                      }
                    }
                  }
                  frame True {
                    # "simulate"
                    n2152 = local read "ON amps"() -> (w3780:dbl)
                    n2153 = local read "OFF amps"() -> (w3781:dbl)
                    n2154 = local read "VOLTS"() -> (w3784:dbl)
                    n2155 = local read "PF"() -> (w3783:dbl)
                    n2156 = Select(t=w3780, s=w3786, f=w3781) -> (s? t:f=w3785:dbl)
                    n2157 = Bundle("OFF amps"=w3785, "VOLTS"=w3784, "PF"=w3783, "OFF amps"=w3785, "VOLTS"=w3784, "PF"=w3783) -> (w3782:T32)  [unwired: 1 in]
                  }
                }
                n2158 = local read "Simulate"() -> (w3740:bool)
                n2159 = stacked-sequence {
                  seq-local: [w3790 _ _ _ _ _ _ _] -> [_ _ _ _ _ _ _ _]
                  seq-local: [w3789 _ _ _ _ _ _ _] -> [_ _ _ _ _ _ _ _]
                  seq-local: [w3788 _ _ _ _ _ _ _] -> [_ _ _ _ _ _ _ w3983]
                  tunnel: w3747 -> [_ w3841 _ _ _ _ _ _]
                  tunnel: w3746 -> [_ _ w3868 _ _ _ _ _]
                  tunnel: w3745 -> [_ _ _ w3896 _ _ _ _]
                  tunnel: w3744 -> [_ _ _ _ w3924 _ _ _]
                  tunnel: w3743 -> [_ _ _ _ _ w3952 _ _]
                  tunnel: w3742 -> [_ _ _ _ _ _ w3980 _]
                  tunnel: w3740 -> [_ _ w3867 w3895 w3923 w3951 w3979 w3985]
                  tunnel: T14 {"1  (A) cal"=1.0, "1 (V) cal"=1.0, "1 (PF) cal"=1.0, "1 (TL) cal"=1.0, "1 (TN) cal"=1.0, "2 (A) cal"=1.0, "2 (V) cal"=1.0, "2 (PF) cal"=1.0, "2 (TL) cal"=1.0, "2 (TN) cal"=1.0} ("CAL LAB01") -> [_ _ w3866 w3894 w3922 w3950 w3978 _]
                  tunnel: w3737 -> [_ _ _ _ _ _ _ w3984]
                  tunnel: w3736 -> [w3793 _ _ _ _ _ _ _]
                  tunnel: w3734 -> [_ w3820 _ _ _ _ _ _]
                  frame #0 {
                    n2160 = Index Array(array=w3793, index=2) -> (element=w3788:bool)
                    n2161 = Index Array(array=w3793, index=1) -> (element=w3789:bool)
                    n2162 = Index Array(array=w3793, index=0) -> (element=w3790:bool)
                    n2163 = local write "Error USB #2"(w3788) -> ()
                    n2164 = local write "Error USB #0"(w3790) -> ()
                    n2165 = local write "Error USB #1"(w3789) -> ()
                    n2166 = stacked-sequence {
                      tunnel: w3790 -> [w3797 _ _ _]
                      tunnel: w3789 -> [_ w3802 _ _]
                      tunnel: 0 -> [w3796 w3801 w3806 _]
                      tunnel: w3788 -> [_ _ w3807 _]
                      frame #0 {
                        n2167 = case shown="True" w3797 {
                          tunnel: w3796 -> [w3798 _]
                          frame False {
                            n2168 = local write "Er USB#0"(w3798) -> ()
                          }
                          frame True {
                            n2169 = local read "Er USB#0"() -> (w3800:dbl)
                            n2170 = Increment(x=w3800) -> (x+1=→"Er USB#0":dbl)
                          }
                        }
                      }
                      frame #1 {
                        n2171 = case shown="True" w3802 {
                          tunnel: w3801 -> [w3803 _]
                          frame False {
                            n2172 = local write "Er USB#1"(w3803) -> ()
                          }
                          frame True {
                            n2173 = local read "Er USB#1"() -> (w3805:dbl)
                            n2174 = Increment(x=w3805) -> (x+1=→"Er USB#1":dbl)
                          }
                        }
                      }
                      frame #2 {
                        n2175 = case shown="True" w3807 {
                          tunnel: w3806 -> [w3808 _]
                          frame False {
                            n2176 = local write "Er USB#2"(w3808) -> ()
                          }
                          frame True {
                            n2177 = local read "Er USB#2"() -> (w3810:dbl)
                            n2178 = Increment(x=w3810) -> (x+1=→"Er USB#2":dbl)
                          }
                        }
                      }
                      frame #3 {
                        w3816 = 10
                        n2179 = local read "Er USB#2"() -> (w3817:dbl)
                        n2180 = local read "Er USB#0"() -> (w3819:dbl)
                        n2181 = local read "Er USB#1"() -> (w3818:dbl)
                        n2182 = Greater Or Equal?(x=w3819, y=w3816) -> (x >= y?=w3814:bool)
                        n2183 = Greater Or Equal?(x=w3818, y=w3816) -> (x >= y?=w3813:bool)
                        n2184 = Greater Or Equal?(x=w3817, y=w3816) -> (x >= y?=w3812:bool)
                        n2185 = Or(x=w3814, y=w3813) -> (x .or. y?=w3815:bool)
                        n2186 = Or(x=w3815, y=w3812) -> (x .or. y?=→"Analog error":bool)
                      }
                    }
                  }
                  frame #1 {
                    # "display graph data on ADM page"
                    n2187 = local write "AI loop time"(w3820) -> ()
                    n2188 = local write "AI"(TRUE) -> ()
                    n2189 = Index Array(array=w3841, index=6) -> (element=→"LAB04-1 (GRAPH)":dynamicdata)
                    n2190 = Index Array(array=w3841, index=7) -> (element=→"LAB04-2 (GRAPH)":dynamicdata)
                    n2191 = Index Array(array=w3841, index=9) -> (element=→"LAB05-2 (GRAPH)":dynamicdata)
                    n2192 = Index Array(array=w3841, index=8) -> (element=→"LAB05-1 (GRAPH)":dynamicdata)
                    n2193 = Index Array(array=w3841, index=5) -> (element=→"LAB03-2 (GRAPH)":dynamicdata)
                    n2194 = Index Array(array=w3841, index=0) -> (element=→"LAB01-1 (GRAPH)":dynamicdata)
                    n2195 = Index Array(array=w3841, index=1) -> (element=→"LAB01-2 (GRAPH)":dynamicdata)
                    n2196 = Index Array(array=w3841, index=2) -> (element=→"LAB02-1 (GRAPH)":dynamicdata)
                    n2197 = Index Array(array=w3841, index=3) -> (element=→"LAB02-2 (GRAPH)":dynamicdata)
                    n2198 = Index Array(array=w3841, index=4) -> (element=→"LAB03-1 (GRAPH)":dynamicdata)
                  }
                  frame #2 {
                    n2199 = case shown="False" w3867 {
                      tunnel: [w3869 w3870] -> w3865
                      tunnel: w3866 -> [_ w3870]
                      frame False {
                        n2200 = local read "CAL LAB01"() -> (w3869:T14)
                      }
                      frame True {
                      }
                    }
